vi "Match number.vi"() -> ()   [LabVIEW 2015]
panel:
  in  "stop":bool
  out "Current Number":u32
  in  "Number to Match":u32
  out "Number of Iterations":i32
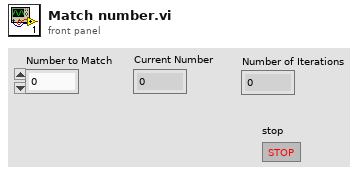
[diagram p1: front panel]
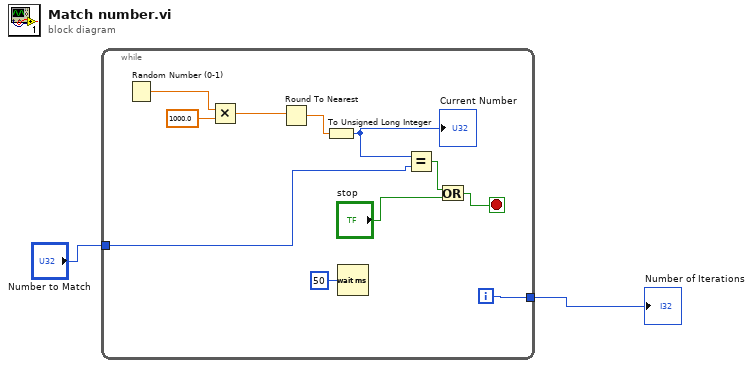
[diagram p0: block diagram]
diagram:
  n1 = while {
    tunnel: [w13] -> w2
    tunnel: "Number to Match" -> [w10]
    i -> [w13]
    stop <- w5 stop-if-true
    n2 = Random Number (0-1) ("Random Number (0-1000)")() -> (number: 0 to 1=w12:dbl)
    n3 = Multiply(x=w12, y=1000.0) -> (x*y=w4:dbl)
    n4 = Round To Nearest(number=w4) -> (nearest integer value=w3:dbl)
    n5 = To Unsigned Long Integer(number=w3) -> (unsigned 32bit integer=w9:u32)
    "Current Number" <- w9
    n6 = Wait (ms)(milliseconds to wait=u32 50) -> ()  [unwired: 1 out]
    n7 = Equal?(x=w9, y=w10) -> (x = y?=w7:bool)
    n8 = Or(x=w7, y="stop") -> (x .or. y?=w5:bool)
  }
  "Number of Iterations" <- w2
